vi "Memory.Pointer.Move Block.Unsafe.vi"(0 "src Pointer in":refnum<class "Memory.Pointer.Void.lvclass">, 1 "length":u64 format="%d bytes", 5 "dst Pointer in":refnum<class "Memory.Pointer.Void.lvclass">, 7 "src offset (0)":u64 format="%d bytes", 9 "dst offset (0)":u64 format="%d bytes", 11 "error in (no error)":errorcluster) -> (4 "src Pointer out":refnum<class "Memory.Pointer.Void.lvclass">, 6 "dst Pointer out":refnum<class "Memory.Pointer.Void.lvclass">, 15 "error out":errorcluster)   [LabVIEW 2016, in "LabVIEW Memory Manager.lvlib" / "Memory.Pointer.Void.lvclass"]
uses:
  Memory.Pointer.Void.lvclass
  Memory.Pointer.Void.lvclass/Memory.Pointer.Void.ctl
  Memory.Pointer.Get Address.vi
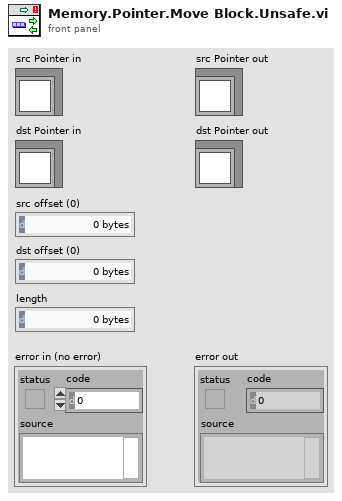
[diagram p1: front panel]
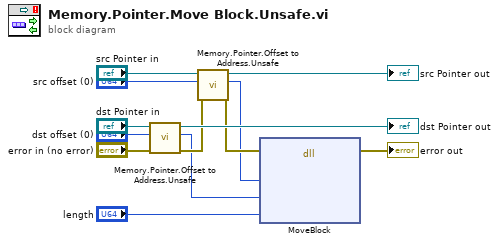
[diagram p0: block diagram]
diagram:
  n1 = call "Memory.Pointer.Offset to Address.Unsafe.vi"("error in (no error)"="error in (no error)", "offset"="dst offset (0)", "Pointer in"="dst Pointer in") -> ("error out"=w11:errorcluster, "address"=w2:u64, "Pointer out"=→"dst Pointer out":refnum<class "Memory.Pointer.Void.lvclass">)  [unwired: 6 in]
  n2 = call "Memory.Pointer.Offset to Address.Unsafe.vi"("error in (no error)"=w11, "offset"="src offset (0)", "Pointer in"="src Pointer in") -> ("error out"=w5:errorcluster, "address"=w1:u64, "Pointer out"=→"src Pointer out":refnum<class "Memory.Pointer.Void.lvclass">)  [unwired: 6 in]
  n3 = dll-call lib="LabVIEW" fn="MoveBlock"(error in=w5, "src"=w1, "dst"=w2, "size"="length") -> (error out=→"error out":errorcluster)  [unwired: 6 in, 1 out]
